vi "demo.vi"() -> ()   [LabVIEW 2014]
uses:
  <vilib>/Plasmionique/MB Master/MB_Master_Serial/MB_Master_Serial.lvclass
panel:
  out "current position":dbl(slide) scale=0.0..95.0
  in  "Band(mm)":dbl=0.1 format="%#_13g"
  in  "Dec(mm/s^2)":dbl=1000.0 format="%#_13g"
  in  "Acc(mm/s^2)":dbl=1000.0 format="%#_13g"
  in  "speed(mm/s)":dbl=100.0 format="%#_13g"
  in  "baud rate (bps)":u32=9600
  in  "VISA Resource":refnum<visa-resource-name>
  in  "stop":bool
  in  "go home":bool
  in  "jog-":bool
  in  "jog+":bool
  in  "position to go":dbl(slide) scale=0.0..95.0
  in  "go":bool
  out "errorCode":i32
  in  "servo":bool=TRUE
  in  "reset error":bool
  in  "axisNo":i32
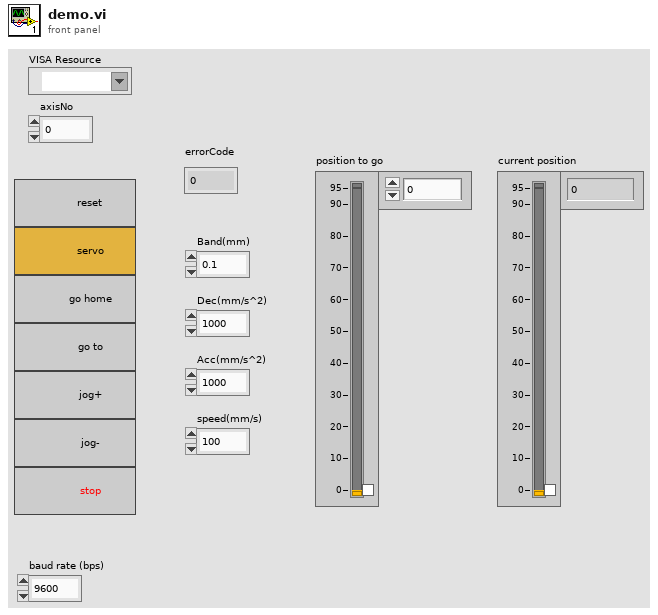
[diagram p1: front panel]
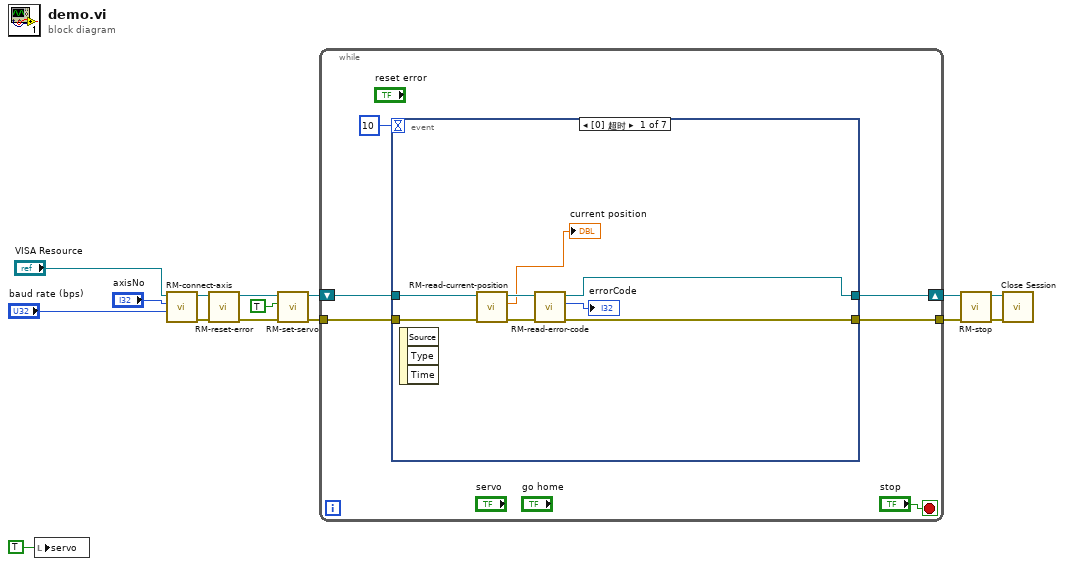
[diagram p0: block diagram]
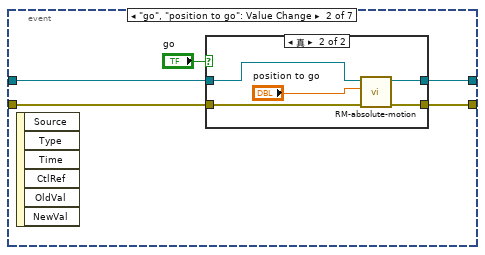
[diagram p2: hidden frame]
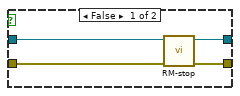
[diagram p3: hidden frame]
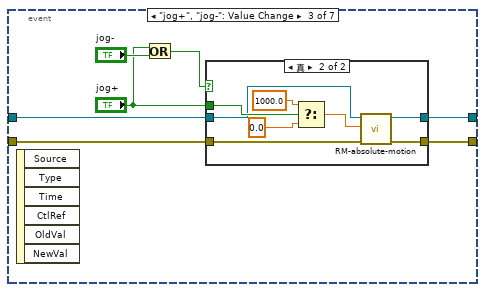
[diagram p4: hidden frame]
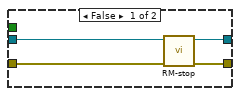
[diagram p5: hidden frame]
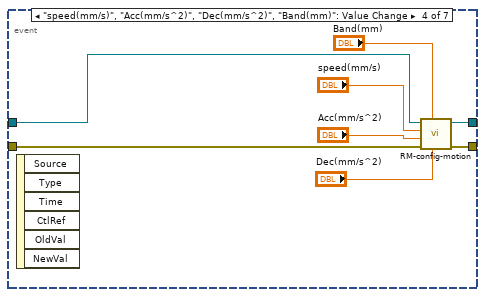
[diagram p6: hidden frame]
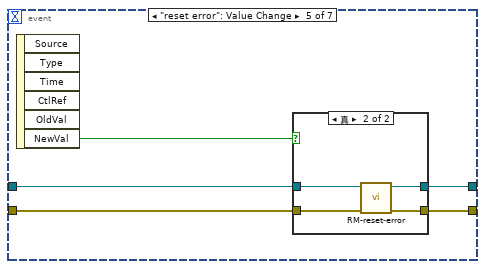
[diagram p7: hidden frame]
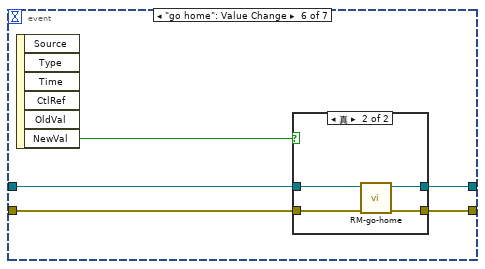
[diagram p9: hidden frame]
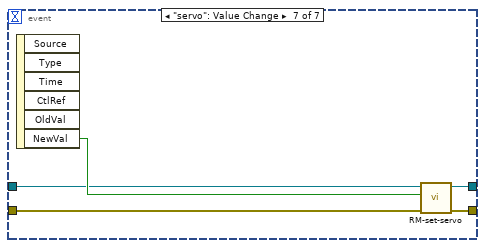
[diagram p11: hidden frame]
diagram:
  n1 = local write "servo"(TRUE ("servo")) -> ()
  n2 = call "RM-connect-axis.vi"("baud rate (bps)"="baud rate (bps)", "axisNo"="axisNo", "VISA引用句柄输入"="VISA Resource") -> ("Error out"=w7:errorcluster, "MB_Master_Serial输出"=w9:refnum<class "MB_Master_Serial.lvclass">)  [unwired: 7 in]
  n3 = call "RM-reset-error.vi"("错误输入（无错误）"=w7, "MB_Master_Serial输入"=w9) -> ("错误输出"=w10:errorcluster, "MB_Master_Serial输出"=w11:refnum<class "MB_Master_Serial.lvclass">)  [unwired: 8 in]
  n4 = call "RM-set-servo.vi"("error in (no error)"=w10, "servo-on?"=TRUE, "MB_Master_Serial输入"=w11) -> ("error out"=w6:errorcluster, "MB_Master_Serial输出"=w8:refnum<class "MB_Master_Serial.lvclass">)  [unwired: 7 in]
  n5 = while {
    shift-right: [w19] -> w5
    shift-left: w8 -> [w20]
    tunnel: [w17] -> w2
    tunnel: w6 -> [w16]
    stop <- "stop" stop-if-true
    n6 = event shown="[0] 超时" {
      selector: _ -> [_ _ _ _ _ _ _]
      dyn-events: _ -> [_ _ _ _ _ _ _]
      timeout: 10 -> [_ _ _ _ _ _ _]
      tunnel: w20 -> [w29 w34 w48 w66 w73 w86 w96]
      tunnel: [w24 w33 w47 w64 w74 w85 w95] -> w19
      tunnel: [w25 w31 w45 w63 w72 w83 w94] -> w17
      tunnel: w16 -> [w28 w30 w46 w65 w71 w82 w93]
      event Timeout {
        n7 = event-data() -> ()  [unwired: 1 in, 3 out]
        n8 = call "RM-read-current-position.vi"("错误输入（无错误）"=w28, "MB_Master_Serial输入"=w29) -> ("错误输出"=w26:errorcluster, "数值"=→"current position":dbl, "MB_Master_Serial输出"=w27:refnum<class "MB_Master_Serial.lvclass">)  [unwired: 7 in]
        n9 = call "RM-read-error-code.vi"("错误输入（无错误）"=w26, "MB_Master_Serial输入"=w27) -> ("错误输出"=w25:errorcluster, "error_code"=→"errorCode":i32, "MB_Master_Serial输出"=w24:refnum<class "MB_Master_Serial.lvclass">)  [unwired: 7 in]
      }
      event "go", "position to go": Value Change {
        n10 = event-data() -> ()  [unwired: 1 in, 6 out]
        n11 = case shown="真" "go" {
          tunnel: w34 -> [w38 w40]
          tunnel: [w37 w42] -> w33
          tunnel: [w35 w41] -> w31
          tunnel: w30 -> [w36 w39]
          frame False {
            n12 = call "RM-stop.vi"("error in (no error)"=w36, "MB_Master_Serial输入"=w38) -> ("error out"=w35:errorcluster, "MB_Master_Serial输出"=w37:refnum<class "MB_Master_Serial.lvclass">)  [unwired: 8 in]
          }
          frame True {
            n13 = call "RM-absolute-motion.vi"("error in (no error)"=w39, "position to go"="position to go", "MB_Master_Serial输入"=w40) -> ("error out"=w41:errorcluster, "MB_Master_Serial输出"=w42:refnum<class "MB_Master_Serial.lvclass">)  [unwired: 7 in]
          }
        }
      }
      event "jog+", "jog-": Value Change {
        n14 = event-data() -> ()  [unwired: 1 in, 6 out]
        n15 = Or(x="jog+", y="jog-") -> (x .or. y?=w49:bool)
        n16 = case shown="真" w49 {
          tunnel: w48 -> [w54 w59]
          tunnel: [w53 w56] -> w47
          tunnel: w46 -> [w52 w58]
          tunnel: [w51 w57] -> w45
          tunnel: "jog+" -> [_ w62]
          frame False {
            n17 = call "RM-stop.vi"("error in (no error)"=w52, "MB_Master_Serial输入"=w54) -> ("error out"=w51:errorcluster, "MB_Master_Serial输出"=w53:refnum<class "MB_Master_Serial.lvclass">)  [unwired: 8 in]
          }
          frame True {
            n18 = Select(t=1000.0, s=w62, f=0.0) -> (s? t:f=w55:dbl)
            n19 = call "RM-absolute-motion.vi"("error in (no error)"=w58, "position to go"=w55, "MB_Master_Serial输入"=w59) -> ("error out"=w57:errorcluster, "MB_Master_Serial输出"=w56:refnum<class "MB_Master_Serial.lvclass">)  [unwired: 7 in]
          }
        }
      }
      event "speed(mm/s)", "Acc(mm/s^2)", "Dec(mm/s^2)", "Band(mm)": Value Change {
        n20 = event-data() -> ()  [unwired: 1 in, 6 out]
        n21 = call "RM-config-motion.vi"("Dec"="Dec(mm/s^2)", "Band"="Band(mm)", "error in (no error)"=w65, "Acc"="Acc(mm/s^2)", "speed"="speed(mm/s)", "MB_Master_Serial输入"=w66) -> ("error out"=w63:errorcluster, "MB_Master_Serial输出"=w64:refnum<class "MB_Master_Serial.lvclass">)  [unwired: 4 in]
      }
      event "reset error": Value Change {
        n22 = event-data() -> ("NewVal"=w75:bool)  [unwired: 1 in, 5 out]
        n23 = case shown="真" w75 {
          tunnel: [w77 w80] -> w74
          tunnel: w73 -> [w77 w81]
          tunnel: [w76 w79] -> w72
          tunnel: w71 -> [w76 w78]
          frame False {
          }
          frame True {
            n24 = call "RM-reset-error.vi"("错误输入（无错误）"=w78, "MB_Master_Serial输入"=w81) -> ("错误输出"=w79:errorcluster, "MB_Master_Serial输出"=w80:refnum<class "MB_Master_Serial.lvclass">)  [unwired: 8 in]
          }
        }
      }
      event "go home": Value Change {
        n25 = event-data() -> ("NewVal"=w84:bool)  [unwired: 1 in, 5 out]
        n26 = case shown="真" w84 {
          tunnel: w86 -> [w88 w92]
          tunnel: [w88 w91] -> w85
          tunnel: [w87 w90] -> w83
          tunnel: w82 -> [w87 w89]
          frame False {
          }
          frame True {
            n27 = call "RM-go-home.vi"("error in (no error)"=w89, "MB_Master_Serial输入"=w92) -> ("error out"=w90:errorcluster, "MB_Master_Serial输出"=w91:refnum<class "MB_Master_Serial.lvclass">)  [unwired: 8 in]
          }
        }
      }
      event "servo": Value Change {
        n28 = event-data() -> ("NewVal"=w97:bool)  [unwired: 1 in, 5 out]
        n29 = call "RM-set-servo.vi"("error in (no error)"=w93, "servo-on?"=w97, "MB_Master_Serial输入"=w96) -> ("error out"=w94:errorcluster, "MB_Master_Serial输出"=w95:refnum<class "MB_Master_Serial.lvclass">)  [unwired: 7 in]
      }
    }
  }
  n30 = call "RM-stop.vi"("error in (no error)"=w2, "MB_Master_Serial输入"=w5) -> ("error out"=w3:errorcluster, "MB_Master_Serial输出"=w4:refnum<class "MB_Master_Serial.lvclass">)  [unwired: 8 in]
  n31 = call-dynamic "Close Session.vi"("error in (no error)"=w3, "MB_Serial session"=w4) -> ()  [unwired: 9 in, 1 out]
